vi "odorStim.vi"(8 "error in (no error)":errorcluster, 10 "Odor #":i32, 11 "Stim in":refnum<class "Stim.lvclass">) -> (0 "error out":errorcluster, 3 "Stim out":refnum<class "Stim.lvclass">)   [LabVIEW 2014]
uses:
  Stim.lvclass
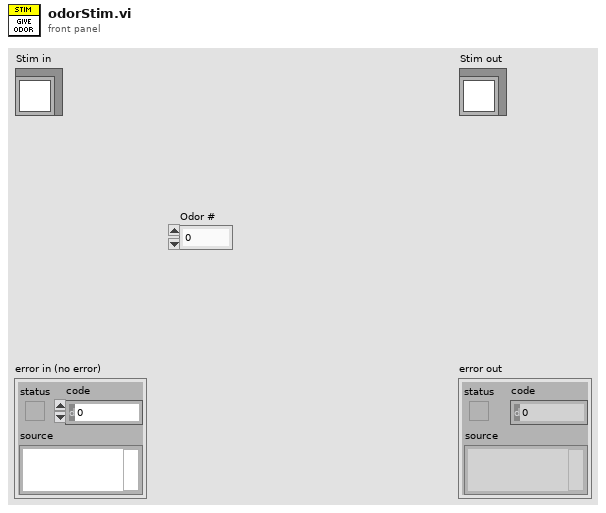
[diagram p1: front panel]
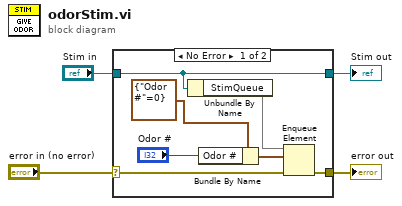
[diagram p0: block diagram]
diagram:
  n1 = case shown="No Error" "error in (no error)" {
    selector: "error in (no error)" -> [w11 w13]
    tunnel: [w10 w13] -> w1
    tunnel: [w9 w12] -> w2
    tunnel: "Stim in" -> [w9 w12]
    frame No Error {
      n2 = Unbundle By Name(w9) -> ("StimQueue"=w8)
      n3 = Bundle By Name(cluster=cluster{"Odor #":i32} {"Odor #"=0} ("element"), "Odor #"="Odor #") -> (w5:cluster{"Odor #":i32})
      n4 = Enqueue Element(queue=w8, element=w5, error in (no error)=w11) -> (error out=w10:errorcluster)  [unwired: 1 in, 2 out]
    }
    frame Error {
    }
  }
  "error out" <- w1
  "Stim out" <- w2
